vi "Release.vi"(8 "error in (no error)":errorcluster, 11 "YP03-60_Y in":refnum<class "YP03-60_Y.lvclass">) -> (0 "error out":errorcluster)   [LabVIEW 2020, in "PowerControl.lvlib" / "YP03-60_Y.lvclass"]
uses:
  YP03-60_Y.lvclass
  YP03-60_X/YP03-60_X.lvclass
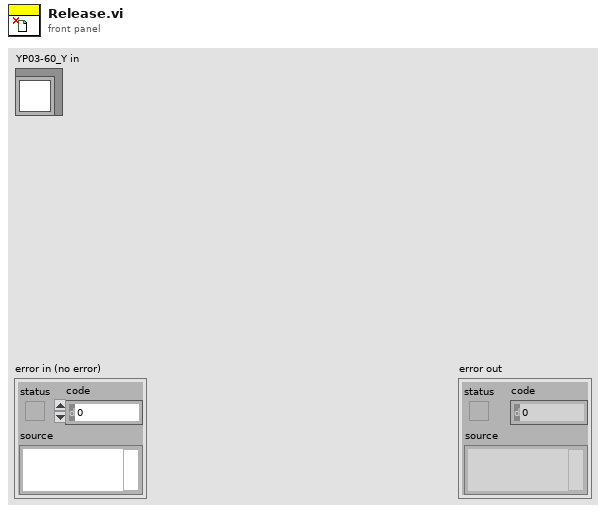
[diagram p1: front panel]
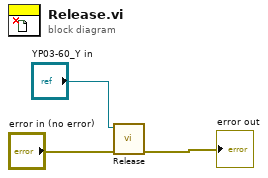
[diagram p0: block diagram]
diagram:
  n1 = call-parent "Release.vi"("error in (no error)"="error in (no error)", "YP03-60_X in"="YP03-60_Y in") -> ("error out"=→"error out":errorcluster)  [unwired: 9 in]
